vi "generate unique file name.vi"(8 "error in":errorcluster, 11 "File in":refnum<class "File.lvclass">) -> (0 "error out":errorcluster, 3 "File out":refnum<class "File.lvclass">)   [LabVIEW 2023, in "File Classes.lvlib" / "File.lvclass"]
uses:
  File.lvclass
  Controls/file operation settings mode.ctl
  File.lvclass/File.ctl
  File Classes.lvlib
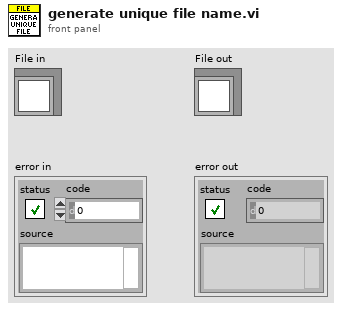
[diagram p1: front panel]
types:
  T1 = typedef "File Classes.lvlib/file operation settings mode.ctl" = enum16{"Copy Files", "Move Files", "Rename Files"}
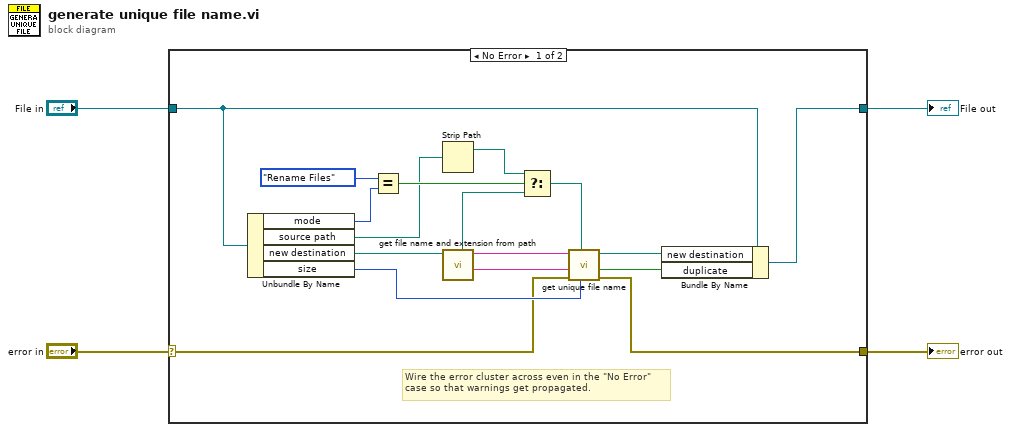
[diagram p0: block diagram]
diagram:
  n1 = case shown="No Error" "error in" {
    selector: "error in" -> [w12 w23]
    tunnel: [w11 w23] -> w3
    tunnel: [w15 w22] -> w1
    tunnel: "File in" -> [w14 w22]
    frame No Error {
      # "Wire the error cluster across even in the \"No Error\"\ncase so that warnings get propagated."
      n2 = Unbundle By Name(w14) -> ("mode"=w20:T1, "source path"=w7:path, "new destination"=w9:path, "size"=w18:i64)
      n3 = Equal?(x=file_operation_settings_mode."Rename Files" ("mode"), y=w20) -> (x = y?=w21:bool)
      n4 = Strip Path(path=w7) -> (stripped path=w6:path)  [unwired: 1 out]
      n5 = call "get file name and extension from path.vi"("fiel path"=w9) -> ("file extension"=w17:string, "file name"=w16:string, "folder path"=w8:path)  [unwired: 8 in]
      n6 = Select(t=w6, s=w21, f=w8) -> (s? t:f=w5:path)
      n7 = call "get unique file name.vi"("size"=w18, "file directory"=w5, "error in"=w12, "file extension"=w17, "file name"=w16) -> ("error out"=w11:errorcluster, "Duplicate?"=w10:bool, "unique file path"=w13:path)  [unwired: 4 in]
      n8 = Bundle By Name(cluster=w14, "new destination"=w13, "duplicate"=w10) -> (w15:refnum<class "File.lvclass">)
    }
    frame Error {
    }
  }
  "error out" <- w3
  "File out" <- w1
